vi "frontEnd.vi"(8 "error in (no error)":errorcluster, 10 "HWControllerEvents":refnum<class "HWControllerEvents.lvclass">, 11 "CameraControlViewer in":refnum<class "CameraControlViewer.lvclass">) -> (0 "error out":errorcluster, 3 "CameraControlViewer out":refnum<class "CameraControlViewer.lvclass">)   [LabVIEW 2009, in "Views.lvlib" / "Camera.lvlib" / "CameraControlViewer.lvclass"]
uses:
  CameraControlViewer.lvclass
  Hal/HWController/HWControllerEvents/HWControllerEvents.lvclass
  CameraControlViewer.lvclass/CameraControlViewer.ctl
panel:
  in  "upload":bool
  in  "stop":bool
  in  "start":bool
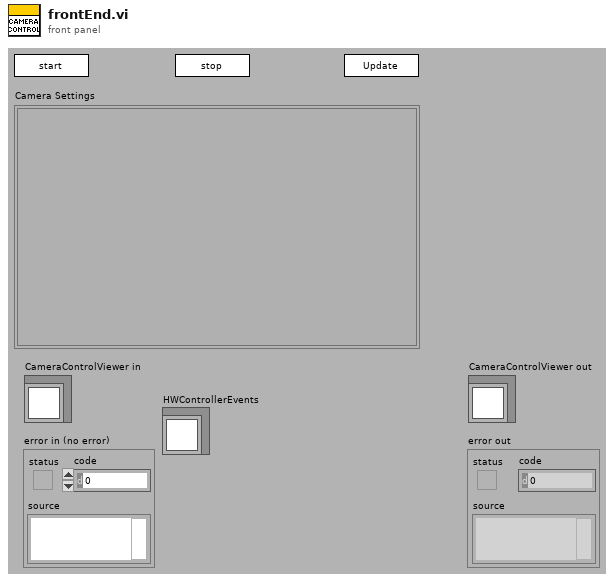
[diagram p1: front panel]
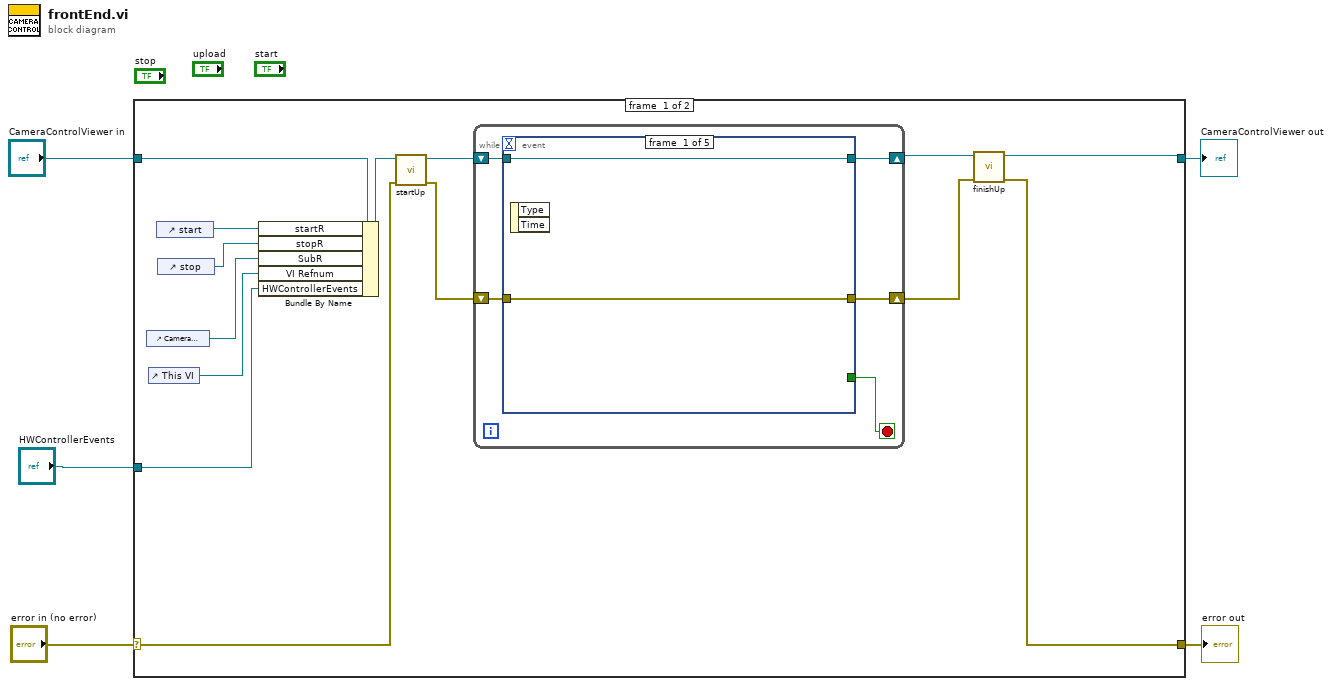
[diagram p0: block diagram]
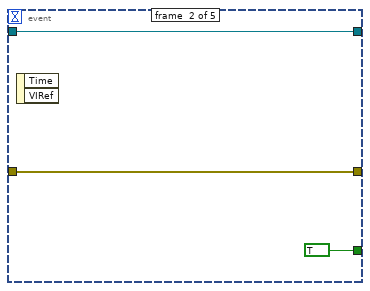
[diagram p2: hidden frame]
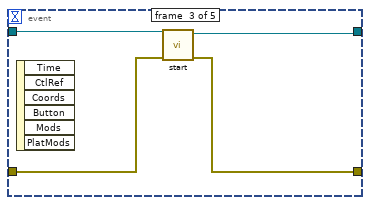
[diagram p3: hidden frame]
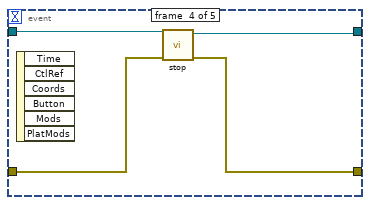
[diagram p4: hidden frame]
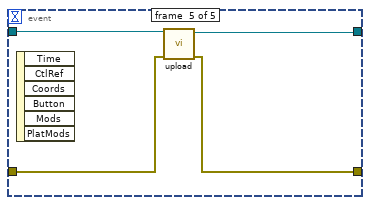
[diagram p5: hidden frame]
diagram:
  n1 = case shown="No Error" "error in (no error)" {
    selector: "error in (no error)" -> [w13 w43]
    tunnel: [w8 w43] -> w4
    tunnel: [w10 w42] -> w2
    tunnel: "CameraControlViewer in" -> [w16 w42]
    tunnel: "HWControllerEvents" -> [w6 _]
    frame #0 {
      n2 = control-ref of="Camera Settings"() -> (w17:refnum<vi>)
      n3 = control-ref of="This VI"() -> (w7:refnum<vi>)
      n4 = control-ref of="start"() -> (w19:refnum<vi>)
      n5 = control-ref of="stop"() -> (w18:refnum<vi>)
      n6 = Bundle By Name(cluster=w16, "startR"=w19, "stopR"=w18, "SubR"=w17, "VI Refnum"=w7, "HWControllerEvents"=w6) -> (w15:refnum<class "CameraControlViewer.lvclass">)
      n7 = call "startUp.vi"("error in (no error)"=w13, "CameraControlViewer in"=w15) -> ("error out"=w12:errorcluster, "CameraControlViewer out"=w14:refnum<class "CameraControlViewer.lvclass">)  [unwired: 8 in]
      n8 = while {
        shift-right: [w23] -> w11
        shift-left: w14 -> [w24]
        shift-right: [w21] -> w9
        shift-left: w12 -> [w22]
        stop <- w20 stop-if-true
        n9 = event shown="[4] \"upload\": Mouse Down" {
          selector: _ -> [_ _ _ _ _]
          dyn-events: _ -> [_ _ _ _ _]
          timeout: _ -> [_ _ _ _ _]
          tunnel: w24 -> [w26 w29 w33 w37 w41]
          tunnel: [w26 w29 w32 w36 w40] -> w23
          tunnel: w22 -> [w25 w28 w31 w35 w39]
          tunnel: [w25 w28 w30 w34 w38] -> w21
          tunnel: [_ TRUE _ _ _] -> w20
          event #0 {
            n10 = event-data() -> ()  [unwired: 1 in, 2 out]
          }
          event #1 {
            n11 = event-data() -> ()  [unwired: 1 in, 2 out]
          }
          event #2 {
            n12 = event-data() -> ()  [unwired: 1 in, 6 out]
            n13 = call "start.vi"("error in (no error)"=w31, "CameraControlViewer in"=w33) -> ("error out"=w30:errorcluster, "CameraControlViewer out"=w32:refnum<class "CameraControlViewer.lvclass">)  [unwired: 8 in]
          }
          event #3 {
            n14 = event-data() -> ()  [unwired: 1 in, 6 out]
            n15 = call "stop.vi"("error in (no error)"=w35, "CameraControlViewer in"=w37) -> ("error out"=w34:errorcluster, "CameraControlViewer out"=w36:refnum<class "CameraControlViewer.lvclass">)  [unwired: 8 in]
          }
          event #4 {
            n16 = event-data() -> ()  [unwired: 1 in, 6 out]
            n17 = call "upload.vi"("error in (no error)"=w39, "CameraControlViewer in"=w41) -> ("error out"=w38:errorcluster, "CameraControlViewer out"=w40:refnum<class "CameraControlViewer.lvclass">)  [unwired: 8 in]
          }
        }
      }
      n18 = call "finishUp.vi"("error in (no error)"=w9, "CameraControlViewer in"=w11) -> ("error out"=w8:errorcluster, "CameraControlViewer out"=w10:refnum<class "CameraControlViewer.lvclass">)  [unwired: 8 in]
    }
    frame #1 {
    }
  }
  "error out" <- w4
  "CameraControlViewer out" <- w2
